vi "Serial Sensor Read.vi"(8 "error in (no error)":errorcluster, 11 "VISA resource name":refnum<visa-resource-name>) -> (0 "error out":errorcluster, 1 "Readings":T1, 2 "appended array":waveform(dbl)[](array[waveform]), 3 "VISA resource name out":refnum<visa-resource-name>)   [LabVIEW 2019]
doc: "This example performs a serial port write and a serial port read. The parameters set for the serial port must match the parameters of the connected instrument or device. The VISA Configure Serial Port VI sets the configuration parameters. The front panel displays the controls used to configure the basic parameters, such as baud rate, data bits, and parity. The VI passes the VISA resource name to other VIs that perform operations on that VISA resource. The VISA Write function sends a command to the serial device and the VISA Read function returns data based on the command. The VISA Close function then closes the reference to the serial device. It is important to close the reference; otherwise, further communication through that port might not be possible."
panel:
  out "Data Output":dbl[](array[numeric])
  # "Serial Sensor Read"
  # "(ppm)"
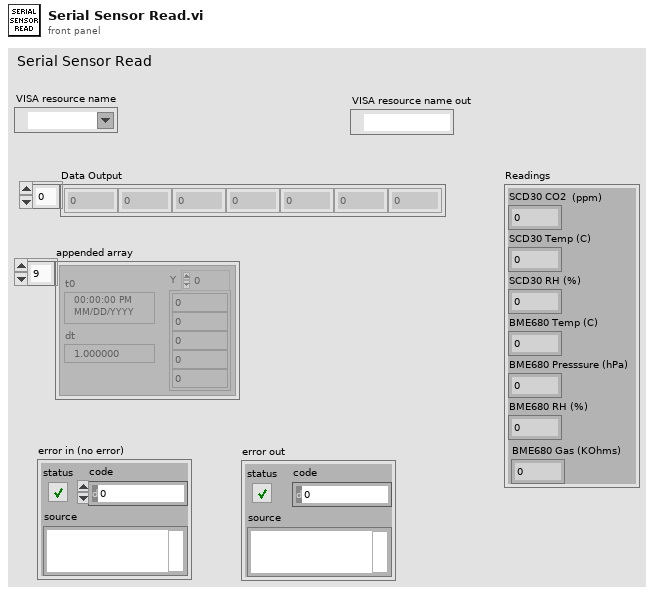
[diagram p1: front panel]
types:
  T1 = cluster{"SCD30 CO2":dbl, "SCD30 Temp (C)":dbl, "SCD30 RH (%)":dbl, "BME680 Temp (C) ":dbl, "BME680 Presssure (hPa)":dbl, "BME680 RH (%) ":dbl, "BME680 Gas (KOhms)":dbl}
  T2 = cluster{"Value":dbl, "Value":dbl, "Value":dbl, "Value":dbl, "Value":dbl, "Value":dbl, "Value":dbl}
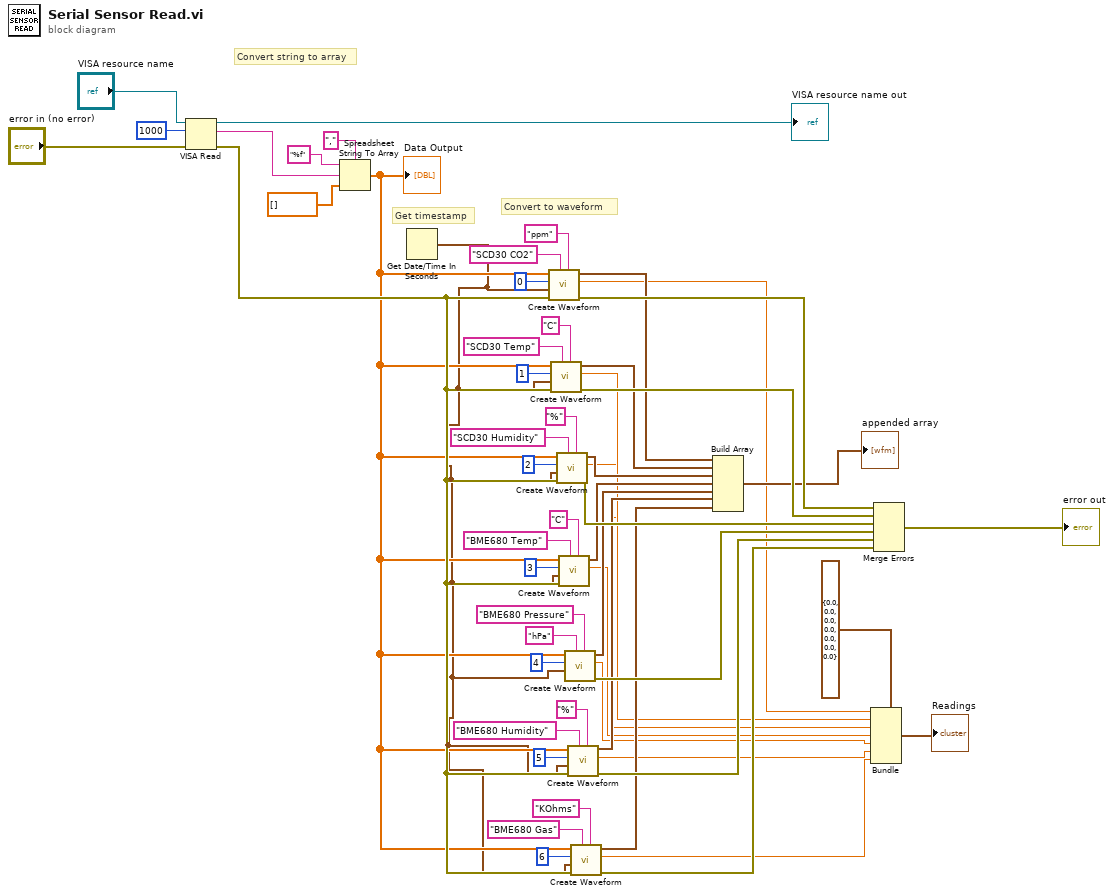
[diagram p0: block diagram]
diagram:
  # "Convert string to array"
  # "Convert to waveform"
  # "Get timestamp"
  n1 = VISA Read(VISA resource name="VISA resource name", byte count=u32 1000, error in (no error)="error in (no error)") -> (VISA resource name out=→"VISA resource name out":refnum<visa-resource-name>, read buffer=w54:string, error out=w29:errorcluster)  [unwired: 1 out]
  n2 = Spreadsheet String To Array(delimiter (Tab)=",", format string="%f", spreadsheet string=w54, array type (2D Dbl)=dbl[] []) -> (array=w14:dbl[])
  "Data Output" <- w14
  n3 = Get Date/Time In Seconds() -> (seconds since 1Jan1904=w1:timestamp)
  n4 = call "Create Waveform.vi"("Unit"="ppm", "Channel name"="SCD30 CO2", "error in (no error)"=w29, "t0"=w1, "index"=0, "array"=w14) -> ("error out"=w28:errorcluster, "Value"=w13:dbl, "output waveform"=w22:waveform(dbl))  [unwired: 3 in]
  n5 = call "Create Waveform.vi"("Unit"="C", "Channel name"="SCD30 Temp", "error in (no error)"=w29, "t0"=w1, "index"=1, "array"=w14) -> ("error out"=w27:errorcluster, "Value"=w12:dbl, "output waveform"=w21:waveform(dbl))  [unwired: 3 in]
  n6 = call "Create Waveform.vi"("Unit"="%", "Channel name"="SCD30 Humidity", "error in (no error)"=w29, "t0"=w1, "index"=2, "array"=w14) -> ("error out"=w26:errorcluster, "Value"=w11:dbl, "output waveform"=w20:waveform(dbl))  [unwired: 3 in]
  n7 = call "Create Waveform.vi"("Unit"="C", "Channel name"="BME680 Temp", "error in (no error)"=w29, "t0"=w1, "index"=3, "array"=w14) -> ("Value"=w10:dbl, "output waveform"=w19:waveform(dbl))  [unwired: 3 in, 1 out]
  n8 = call "Create Waveform.vi"("Unit"="BME680 Pressure", "Channel name"="hPa", "t0"=w1, "index"=4, "array"=w14) -> ("error out"=w25:errorcluster, "Value"=w9:dbl, "output waveform"=w18:waveform(dbl))  [unwired: 4 in]
  n9 = call "Create Waveform.vi"("Unit"="%", "Channel name"="BME680 Humidity", "error in (no error)"=w29, "t0"=w1, "index"=5, "array"=w14) -> ("error out"=w24:errorcluster, "Value"=w8:dbl, "output waveform"=w17:waveform(dbl))  [unwired: 3 in]
  n10 = call "Create Waveform.vi"("Unit"="KOhms", "Channel name"="BME680 Gas", "error in (no error)"=w29, "t0"=w1, "index"=6, "array"=w14) -> ("error out"=w23:errorcluster, "Value"=w7:dbl, "output waveform"=w16:waveform(dbl))  [unwired: 3 in]
  n11 = Build Array(w22, w21, w20, w19, w18, w17, w16) -> (→"appended array":waveform(dbl)[])
  n12 = Bundle(cluster=T2 {"Value"=0.0, "Value"=0.0, "Value"=0.0, "Value"=0.0, "Value"=0.0, "Value"=0.0, "Value"=0.0}, "Value"=w13, "Value"=w12, "Value"=w11, "Value"=w10, "Value"=w9, "Value"=w8, "Value"=w7) -> (→"Readings":T2)
  n13 = Merge Errors(w28, w27, w26, w25, w24, w23) -> (→"error out":errorcluster)
